vi "State8-Reverse.vi"(11 "Numeric":dbl) -> (1 "Cluster":T1, 2 "Front/Back 2":enum16{"Forward", "Backward", "Stop"}(ring), 3 "Left/Right":enum16{"Left", "Right", "Stop"}(ring), 4 "Enum":T2, 5 "Left/Right Speed":u32)   [LabVIEW 2014]
uses:
  FPGA Bitfiles/Parking States.ctl
  FPGA Bitfiles/Parking States Indicators.ctl
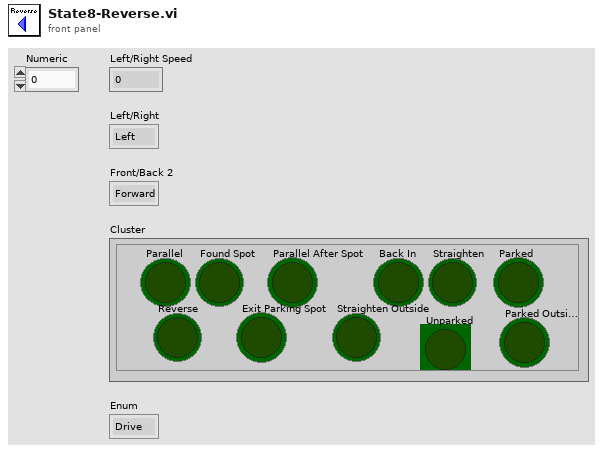
[diagram p1: front panel]
types:
  T1 = typedef "Parking States Indicators.ctl" = cluster{"Parallel":bool, "Found Spot":bool, "Parallel After Spot":bool, "Back In":bool, "Straighten":bool, "Parked":bool, "Reverse":bool, "Exit Parking Spot":bool, "Straighten Outside":bool, "Unparked":bool, "Parked Outside":bool}
  T2 = typedef "Parking States.ctl" = enum16{"Drive", "Parallel", "Found Spot", "Parallel After Spot", "Back In", "Straighten", "Parked", "Reverse", "Exit Parking Spot", "Straighten Outside", "Unparked", "Parked Outside"}
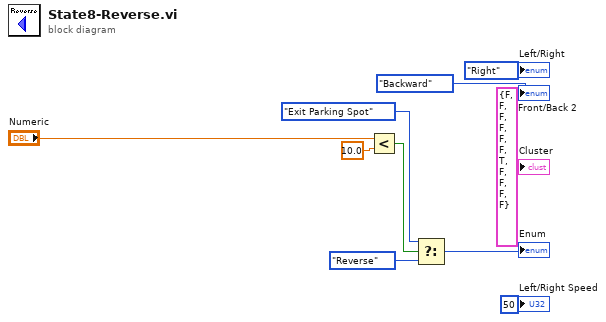
[diagram p0: block diagram]
diagram:
  n1 = Less?(x="Numeric", y=10.0) -> (x < y?=w4:bool)
  n2 = Select(t=Parking_States."Exit Parking Spot", s=w4, f=Parking_States."Reverse") -> (s? t:f=→"Enum":T2)
  "Cluster" <- T1 {"Parallel"=FALSE, "Found Spot"=FALSE, "Parallel After Spot"=FALSE, "Back In"=FALSE, "Straighten"=FALSE, "Parked"=FALSE, "Reverse"=TRUE, "Exit Parking Spot"=FALSE, "Straighten Outside"=FALSE, "Unparked"=FALSE, "Parked Outside"=FALSE} ("Cluster")
  "Left/Right Speed" <- u32 50 ("Left/Right Speed")
  "Front/Back 2" <- enum16{"Forward", "Backward", "Stop"}."Backward" ("Front/Back 2")
  "Left/Right" <- enum16{"Left", "Right", "Stop"}."Right" ("Left/Right")
